vi "demo_DeepLTK GPU by NGENE.vi"(11 "Stop Demo":refnum<user-event>) -> ()   [LabVIEW 2020]
panel:
  # "PROVIDING COMPLETE TOOLCHAIN FOR DEEP LEARNING SYSTEMS\n\nDevelop custom and efficient deep learning models including data collection and annotation with NNotate, deep neural network training and optimization with DeepLTK, as well as deployment for inference on different hardware platforms such as embedded CPUs, GPUs and FPGAs. \nhttps://www.ngene.co/"
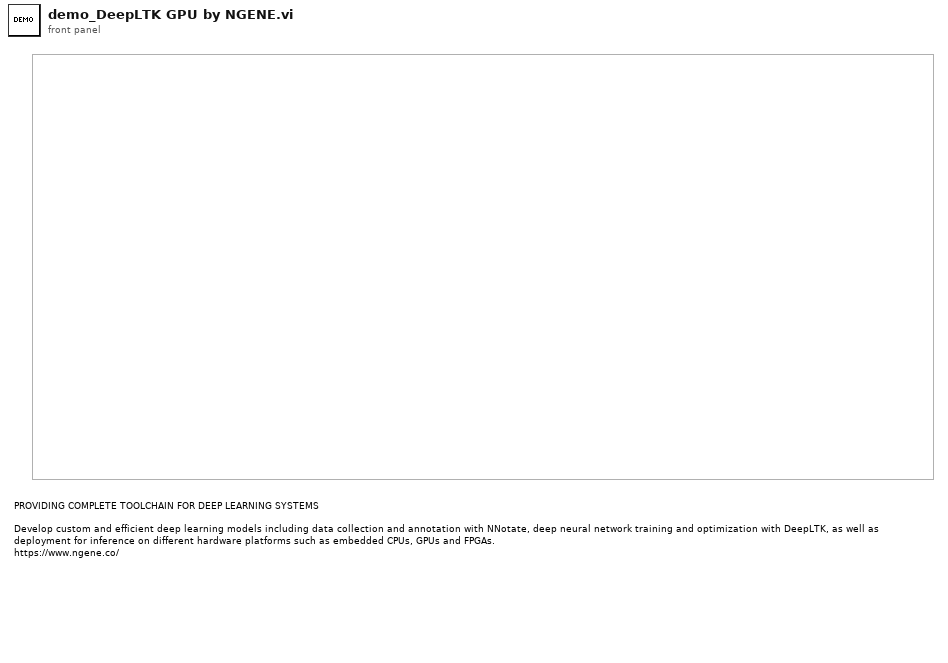
[diagram p1: front panel]
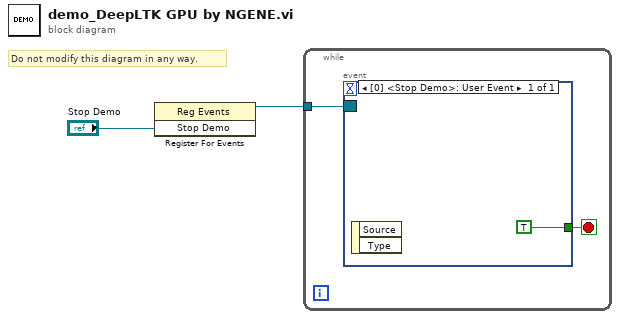
[diagram p0: block diagram]
diagram:
  # "Do not modify this diagram in any way."
  n1 = register-events("Stop Demo") -> (reference out=w1:refnum<event-registration>)  [unwired: 2 in, 1 out]
  n2 = while {
    tunnel: w1 -> [w4]
    stop <- w3 stop-if-true
    n3 = event shown="[0] <Stop Demo>: User Event" {
      selector: w4 -> [_]
      dyn-events: _ -> [_]
      timeout: _ -> [_]
      tunnel: [TRUE] -> w3
      event User Event {
        n4 = event-data() -> ()  [unwired: 1 in, 2 out]
      }
    }
  }
